vi "Generate Temporary File Path.vi"(8 "error in (no error)":errorcluster, 10 "Temporary File Extension (tmp)":string="tmp") -> (0 "error out":errorcluster, 3 "Unique Temporary File Path":path)   [LabVIEW 2020]
doc: "Returns a unique file path to the temporary directory. This VI only returns a path. It does not create the temporary file."
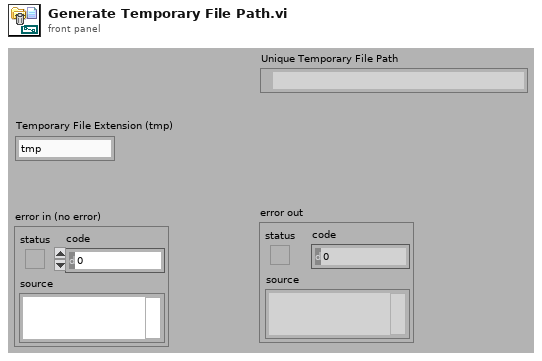
[diagram p1: front panel]
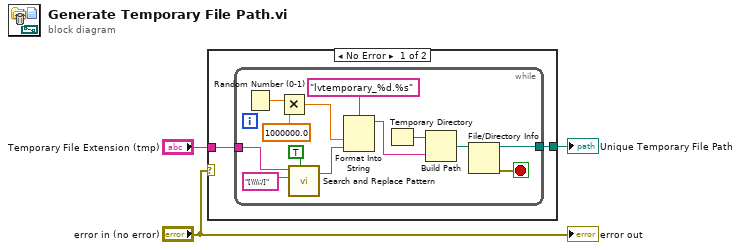
[diagram p0: block diagram]
diagram:
  n1 = case shown="No Error" "error in (no error)" {
    tunnel: "Temporary File Extension (tmp)" -> [w5 _]
    tunnel: [w4 _] -> w1
    frame No Error {
      n2 = while {
        tunnel: w5 -> [w9]
        tunnel: [w10] -> w4
        stop <- w11 stop-if-true
        n3 = Random Number (0-1)() -> (number: 0 to 1=w18:dbl)
        n4 = Multiply(x=w18, y=1000000.0) -> (x*y=w15:dbl)
        n5 = call "Search and Replace Pattern.vi"("string"=w9, "regular expression (\"\")"="[\\\\:/]" ("regular expression (\"\")"), "replace all? (F)"=TRUE) -> ("result string"=w8:string)  [unwired: 1 in, 2 out]
        n6 = Format Into String(format string="lvtemporary_%d.%s", w15, w8) -> (resulting string=w14:string)  [unwired: 2 in, 1 out]
        n7 = Temporary Directory() -> (w13:path)
        n8 = Build Path(base path=w13, name or relative path=w14) -> (appended path=w12:path)
        n9 = File/Directory Info(path=w12) -> (path out=w10:path, error out=w11:errorcluster)  [unwired: 1 in, 5 out]
      }
    }
    frame Error {
    }
  }
  "Unique Temporary File Path" <- w1
  "error out" <- "error in (no error)"
